vi "Daq_vs_Keithley.vi"() -> ()   [LabVIEW 2015]
uses:
  <vilib>/Utility/error.llb/DialogType.ctl
  <vilib>/DAQmx/read.llb/DAQmx Read (Analog Wfm 1Chan NSamp).vi
  <vilib>/Analysis/baseanly.llb/Mean (DBL).vi
  <vilib>/DAQmx/create/channels.llb/DAQmx Create Channel (AI-Voltage-Basic).vi
  <vilib>/DAQmx/configure/timing.llb/DAQmx Timing (Sample Clock).vi
  <vilib>/DAQmx/miscellaneous.llb/DAQmx Fill In Error Info.vi
  <vilib>/Analysis/NI_AALBase.lvlib
panel:
  in  "n":i8
  out "Lag":dbl
  out "standard deviation 2":dbl format="%0.6f"
  out "standard deviation":dbl format="%0.6f"
  in  "IV converter":refnum<visa-resource-name>="GPIB0::20::INSTR"
  out "Waveform Chart":cluster{"mean":dbl, dbl}(graph)
  in  "stop":bool
  out "Waveform Graph":waveform(dbl)(graph)
  in  "Number of Samples":i32=100
  in  "Sample Rate":dbl=1000.0
  in  "Terminal Configuration":i32(ring)=-1 items=["default"=-1, "RSE"=10083, "NRSE"=10078, "Differential"=10106, "Pseudodifferential"=12529]
  in  "Max Voltage":dbl=5.0
  in  "Min Voltage":dbl=-5.0
  in  "Physical Channel":tag="Dev1/ai0"
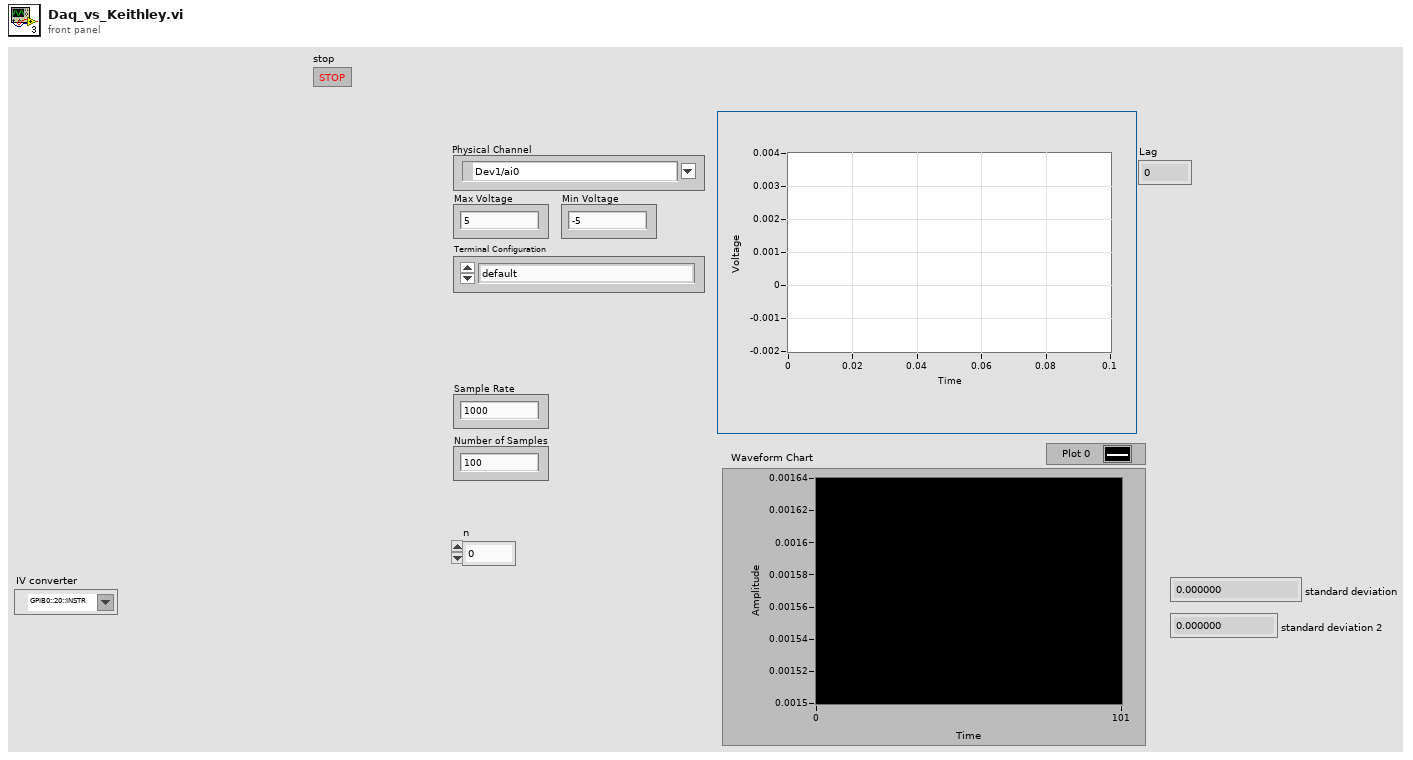
[diagram p1: front panel]
types:
  T1 = typedef "DialogType.ctl" = u16
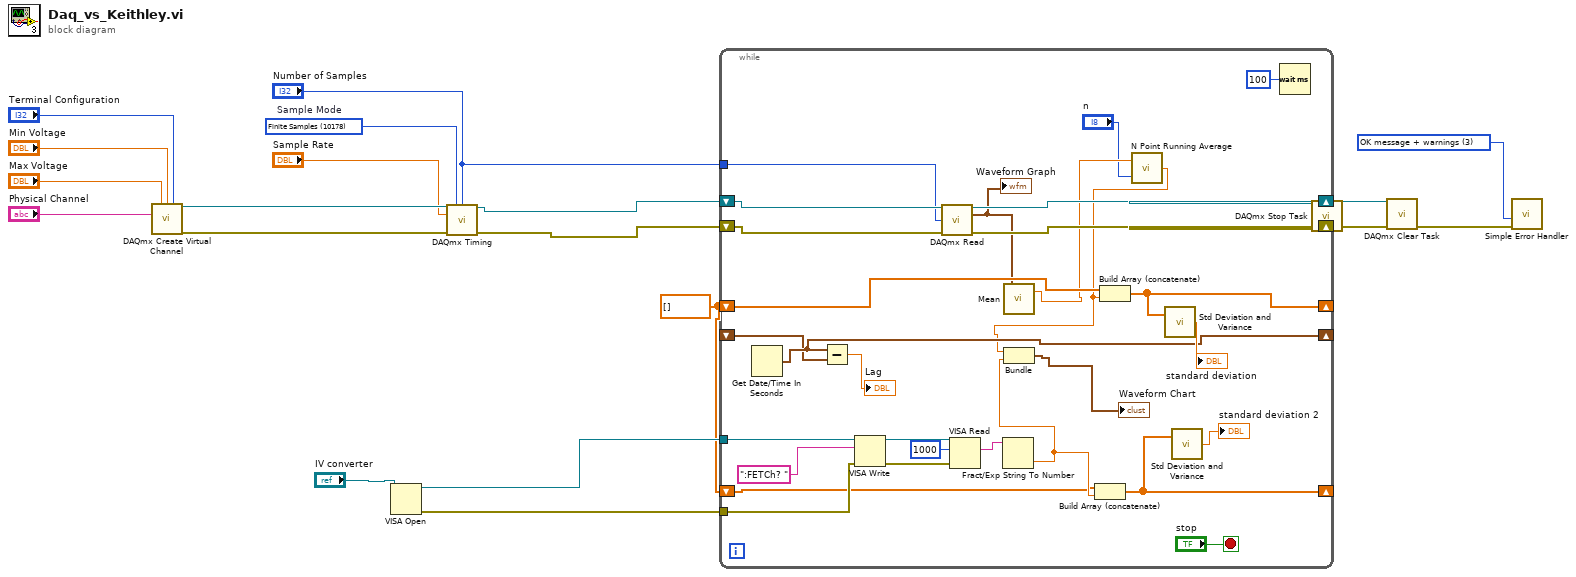
[diagram p0: block diagram]
diagram:
  w1 = dbl[] []
  w8 = T1 3 items=["no dialog", "OK message", "continue or stop message", "OK message + warnings", "continue/stop + warnings"] ("type of dialog (OK msg:1)")
  w21 = 10178 items=["Finite Samples"=10178, "Continuous Samples"=10123, "Hardware Timed Single Point"=12522]  # Sample Mode
  n1 = call-poly <vilib>:"DAQmx Create Virtual Channel.vi"("maximum value"="Max Voltage", "minimum value"="Min Voltage", "input terminal configuration"="Terminal Configuration", "physical channels"="Physical Channel") -> ("task out"=w19:refnum<k21>, "error out"=w20:errorcluster)  [unwired: 10 in]
  n2 = VISA Open(VISA resource name="IV converter") -> (VISA resource name=w3:refnum<visa-resource-name>, error out=w2:errorcluster)  [unwired: 4 in]
  n3 = call-poly <vilib>:"DAQmx Timing.vi"("task/channels in"=w19, "sample mode"=w21, "samples per channel"="Number of Samples", "rate"="Sample Rate", "error in"=w20) -> ("task out"=w6:refnum<k21>, "error out"=w5:errorcluster)  [unwired: 9 in]
  n4 = while {
    shift-right: [w50] -> w10
    shift-left: w6 -> [w47]
    shift-right: [w49] -> w9
    shift-left: w5 -> [w46]
    tunnel: "Number of Samples" -> [w45]
    tunnel: w3 -> [w40]
    tunnel: w2 -> [w39]
    shift-right: [w25] -> _
    shift-left: w1 -> [w36]
    shift-right: [w32] -> _
    shift-left: w1 -> [w33]
    shift-right: [w30] -> _
    shift-left: _ -> [w29]
    stop <- "stop" stop-if-true
    n5 = Get Date/Time In Seconds() -> (seconds since 1Jan1904=w30:timestamp)
    n6 = Subtract(x=w30, y=w29) -> (x-y=→"Lag":dbl)
    n7 = VISA Write(VISA resource name=w40, write buffer=":FETCh? " ("data"), error in (no error)=w39) -> (VISA resource name out=w42:refnum<visa-resource-name>, error out=w41:errorcluster)  [unwired: 1 out]
    n8 = call-poly <vilib>:"DAQmx Read.vi"("task/channels in"=w47, "number of samples per channel"=w45, "error in"=w46) -> ("task out"=w50:refnum<k21>, "data"=w27:waveform(dbl), "error out"=w49:errorcluster)  [unwired: 10 in]
    "Waveform Graph" <- w27
    n9 = VISA Read(VISA resource name=w42, byte count=u32 1000, error in (no error)=w41) -> (read buffer=w37:string)  [unwired: 3 out]
    n10 = Fract/Exp String To Number(string=w37) -> (number=w34:dbl)  [unwired: 3 in, 1 out]
    n11 = call-poly <vilib>:"Mean.vi"("X"=w27) -> ("mean"=w26:dbl)  [unwired: 1 out]
    n12 = Build Array (concatenate)(w33, w34) -> (w32:dbl[])
    n13 = call "N Point Running Average.vi"("n"="n", "Input"=w26) -> ("Output"=w23:dbl)
    n14 = Bundle("Output"=w23, w34) -> (→"Waveform Chart":cluster{"Output":dbl, dbl})  [unwired: 1 in]
    n15 = Build Array (concatenate)(w36, w23) -> (w25:dbl[])
    n16 = call <vilib>:"Std Deviation and Variance.vi"("X"=w25) -> ("standard deviation"=→"standard deviation":dbl)  [unwired: 1 in, 2 out]
    n17 = call <vilib>:"Std Deviation and Variance.vi"("X"=w32) -> ("standard deviation"=→"standard deviation 2":dbl)  [unwired: 1 in, 2 out]
    n18 = Wait (ms)(milliseconds to wait=u32 100) -> ()  [unwired: 1 out]
  }
  n19 = call <vilib>:"DAQmx Stop Task.vi"("task/channels in"=w10, "error in"=w9) -> ("task out"=w12:refnum<k21>, "error out"=w11:errorcluster)  [unwired: 12 in]
  n20 = call <vilib>:"DAQmx Clear Task.vi"("task in"=w12, "error in"=w11) -> ("error out"=w18:errorcluster)  [unwired: 13 in]
  n21 = call <vilib>:"Simple Error Handler.vi"("type of dialog (OK msg:1)"=w8, "error in (no error)"=w18) -> ()  [unwired: 3 in, 5 out]
